vi "WAPIAerPosgrabReadIndex.vi"(9 "error in (no error)":errorcluster) -> (2 "index":i32, 6 "error out":errorcluster)   [LabVIEW 2009]
uses:
  win50032.dll
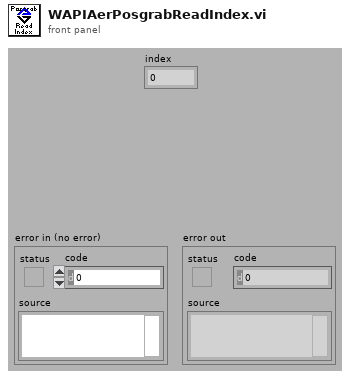
[diagram p1: front panel]
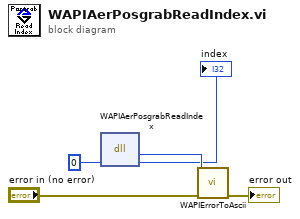
[diagram p0: block diagram]
diagram:
  n1 = dll-call lib="Win50032.dll" fn="WAPIAerPosgrabReadIndex"("index"=0 ("size")) -> ("return type"=w5:u32, "index"=→"index":i32)  [unwired: 3 in, 2 out]
  n2 = call "WAPIErrorToAscii.vi"("error in (no error)"="error in (no error)", "error"=w5) -> ("error out"=→"error out":errorcluster)  [unwired: 8 in, 1 out]
